vi "Read Skip when tabbing.vi"(8 "error in (no error)":errorcluster, 11 "String dropdown D Element in":refnum<class "String dropdown D Element.lvclass">) -> (0 "error out":errorcluster, 2 "Skip when tabbing":bool, 3 "String dropdown D Element out":refnum<class "String dropdown D Element.lvclass">)   [LabVIEW 2018, in "D Datagrid Library.lvlib" / "String dropdown D Element.lvclass"]
uses:
  String dropdown D Element.lvclass
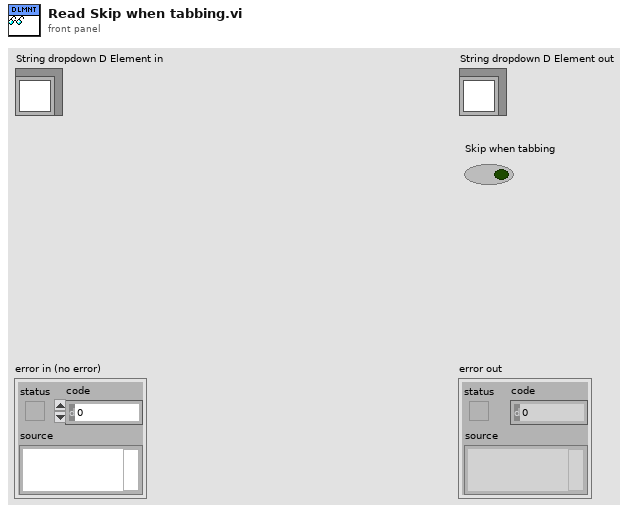
[diagram p1: front panel]
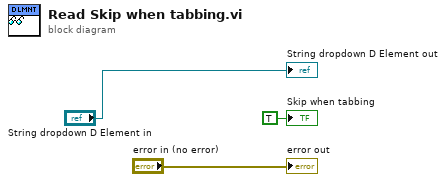
[diagram p0: block diagram]
diagram:
  "error out" <- "error in (no error)"
  "String dropdown D Element out" <- "String dropdown D Element in"
  "Skip when tabbing" <- TRUE ("Skip when tabbing")
